vi "WhileLoopDOBlink.vi"() -> ()   [LabVIEW 2020]
uses:
  <instrlib>/HandsOnPi2040/cti-drivers-lv-visa-main/CTI-Visa/Identity.ctl
  <instrlib>/HandsOnPi2040/Public/DigOuts.ctl
  <instrlib>/HandsOnPi2040/HandsOnPi2040.lvlib
  <instrlib>/HandsOnPi2040/cti-drivers-lv-visa-main/CTI-Visa/CTI-Visa.lvlib
panel:
  out "Identity":T1
  out "error out":errorcluster
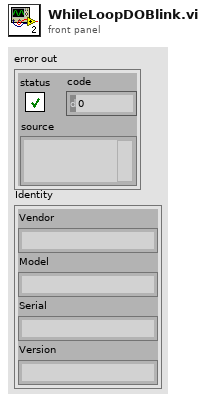
[diagram p1: front panel]
types:
  T1 = typedef "CTI-Visa.lvlib/Identity.ctl" = cluster{"Vendor":string, "Model":string, "Serial":string, "Version":string}
  T2 = typedef "HandsOnPi2040.lvlib/DigOuts.ctl" = enum16{"No DO - Error", "DO1 (GPIO2)", "DO2 (GPIO3)", "DO3 (GPIO4)", "DO4 (GPIO5)", "BEEP (GPIO6)"}
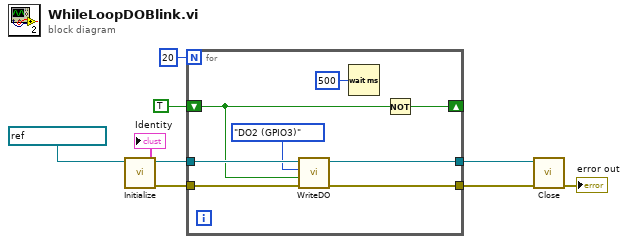
[diagram p0: block diagram]
diagram:
  n1 = call <instrlib>:"Initialize.vi"("VISA resource name"=refnum<visa-resource-name> "ASRL5::INSTR") -> ("error out"=w9:errorcluster, "Identity"=→"Identity":T1, "VISA resource name out"=w6:refnum<visa-resource-name>)  [unwired: 8 in]
  n2 = for {
    N: 20 -> [_]
    tunnel: w9 -> [w17]
    tunnel: [w16] -> w8
    tunnel: [w15] -> w7
    tunnel: w6 -> [w14]
    shift-right: [w13] -> _
    shift-left: TRUE -> [w12]
    n3 = call <instrlib>:"WriteDO.vi"("error in (no error)"=w17, "DO Value (True)"=w12, "Output"=DigOuts."DO2 (GPIO3)", "VISA resource name"=w14) -> ("error out"=w16:errorcluster, "VISA resource name out"=w15:refnum<visa-resource-name>)  [unwired: 6 in]
    n4 = Wait (ms)(milliseconds to wait=u32 500) -> ()  [unwired: 1 out]
    n5 = Not(x=w12) -> (.not. x?=w13:bool)
  }
  n6 = call <instrlib>:"Close.vi"("error in (no error)"=w8, "VISA resource name"=w7) -> ("error out"=→"error out":errorcluster)  [unwired: 9 in]
